vi "ackIRQ.vi"(8 "error in (no error)":errorcluster, 11 "ComponentData in":refnum<class "ComponentData.lvclass">) -> (0 "error out":errorcluster, 3 "ComponentData out":refnum<class "ComponentData.lvclass">)   [LabVIEW 2013, in "ComponentData.lvlib" / "ComponentData.lvclass"]
uses:
  <userlib>/Common/Component/Application/RT/ComponentData/ComponentData/ComponentData.lvclass
  <userlib>/Common/Component/Application/RT/ComponentData/ComponentData/ComponentData.lvclass/ComponentData.ctl
  <userlib>/Common/Component/Application/RT/ComponentData/IRQHandler/IRQHandler.lvclass
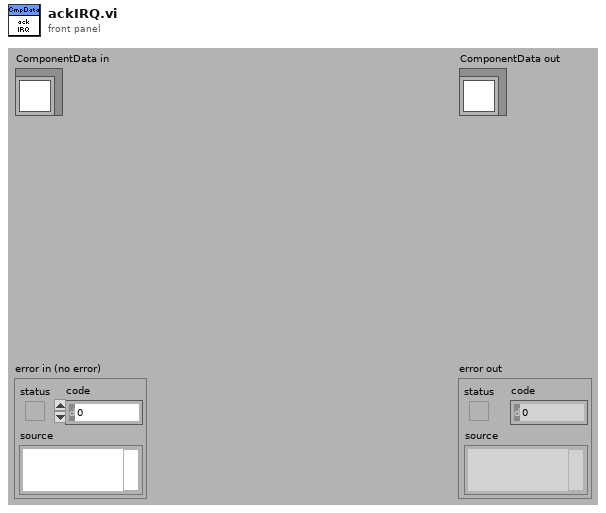
[diagram p1: front panel]
types:
  T1 = typedef "ComponentData.lvlib/fpgaVIRefCRIO9074.ctl" = refnum<k20>
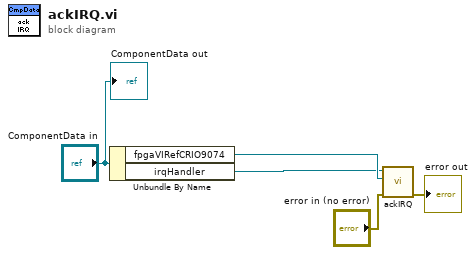
[diagram p0: block diagram]
diagram:
  n1 = Unbundle By Name("ComponentData in") -> ("fpgaVIRefCRIO9074"=w2:T1, "irqHandler"=w1:refnum<class "IRQHandler.lvclass">)
  n2 = call <userlib>:"ackIRQ.vi"("error in (no error)"="error in (no error)", "fpgaVIRefCRIO9074"=w2, "IRQHandler in"=w1) -> ("error out"=→"error out":errorcluster)  [unwired: 7 in, 1 out]
  "ComponentData out" <- "ComponentData in"
